vi "Start DIO Tasks.vi"(8 "error in (no error)":errorcluster) -> (0 "error out":errorcluster)   [LabVIEW 2013]
doc: "This sub-VI initializes necessary digital and analog I/O tasks for the table and pressure control system."
uses:
  Globals/DIO_task_array.vi
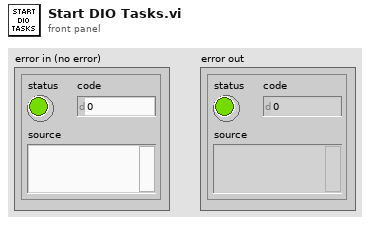
[diagram p1: front panel]
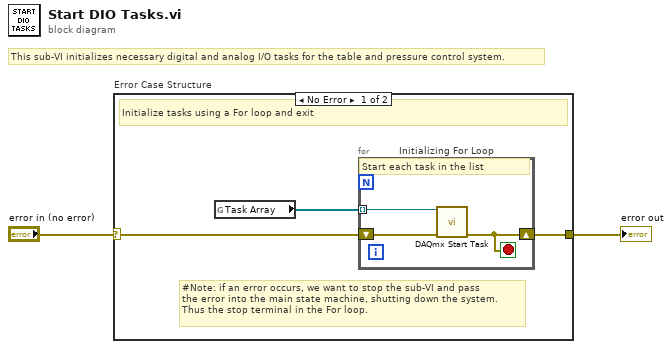
[diagram p0: block diagram]
diagram:
  # "This sub-VI initializes necessary digital and analog I/O tasks for the table and pressure control system."
  n1 = case "Error Case Structure" shown="No Error" "error in (no error)" {
    selector: "error in (no error)" -> [w4 w9]
    tunnel: [w5 w9] -> w2
    frame No Error {
      # "#Note: if an error occurs, we want to stop the sub-VI and pass\nthe error into the main state machine, shutting down the system.\nThus the stop terminal in the For loop."
      # "Initialize tasks using a For loop and exit"
      n2 = global read "DIO_task_array.vi" "Task Array"() -> (w3:refnum<k21>[])
      n3 = for "Initializing For Loop" {
        tunnel: w3 -> [w6] mode=indexing
        shift-right: [w7] -> w5
        shift-left: w4 -> [w8]
        stop <- w7 stop-if-true
        # "Start each task in the list"
        n4 = call <vilib>:"DAQmx Start Task.vi"("task/channels in"=w6, "error in"=w8) -> ("error out"=w7:errorcluster)  [unwired: 12 in, 1 out]
      }
    }
    frame Error {
      # "Pass through and exit without intializing"
    }
  }
  "error out" <- w2
